vi "HOST_MAIN.vi"() -> ()   [LabVIEW 2023]
uses:
  RT/Type/Type_TCP_Cmd.ctl
  HOST_GLOBAL.vi
panel:
  in  "Bool_Exit":bool
  in  "Bool_main":bool
  in  "Bool_Config":bool
  out "Tab_Main":enum32{"Main", "Config"}(tab)
  out "Connected":i32(slide) scale=0.0..10.0
  out "R_GCP":sgl(slide) scale=0.0..100.0
  out "L_GCP":sgl(slide) scale=0.0..100.0
  in  "Save Data Path":path=path "C:/DataSave/Exosuit_FFM"
  out "TCP Connected":bool
  out "R_Velocity":sgl caption="[ kN ]" format="%#.4f"
  out "R_Position":sgl caption="[ kN ]" format="%#.4f"
  out "L_Velocity":sgl caption="[ kN ]" format="%#.4f"
  out "L_Position":sgl caption="[ kN ]" format="%#.4f"
  out "R_LOAD":sgl caption="[ N ]" format="%#.2f"
  out "L_LOAD":sgl caption="[ N ]" format="%#.2f"
  out "R_THIGH":sgl caption="[ kN ]"
  out "L_THIGH":sgl caption="[ kN ]"
  out "Pos_Chart":sgl[][](graph) caption="Motor Position"
  out "Load_Chart":sgl[][](graph) caption="LoadCell"
  out "IMU_Chart":sgl[][](graph) caption="IMU Sensor ROLL"
  in  "Bool_Auto_Stop":bool
  in  "Bool_Auto_Start":bool
  in  "Bool_SendConfig":bool
  in  "Param":T1={"Common"={"Velocity range"={"output high"=29.0, "output low"=-29.0}, "Vel_BasePos"=5, "Ref.Load_FindBase_L"=2.0, "Ref.Load_FindBase_R"=2.0, "Force_Peak"=150.0}, "Param_Left"={"L_기준값"=90.0, "L_검출값"=120.0, "L_End %"=42, "L_Onset %"=4, "L_Peak %"=28, "L_Pos"=0, "L_Offset"=0.0}, "Param_Right"={"R_기준값"=90.0, "R_검출값"=120.0, "R_End %"=42, "R_Onset %"=4, "R_Peak %"=28, "R_Pos"=0, "R_Offset"=0.0}}
  in  "탭 컨트롤":enum32{"Sensor", "Motor Status"}(tab)
  out "RIGHT":T2
  out "LEFT":T3
  in  "Port Number":u16
  in  "IP Address":string
  in  "Bool_Save_Config":bool
  # "실시간 보행 보조 로봇 모니터링 소프트웨어"
  # "Copyright ⓒ 2019 CAU all rights reserved"
  # "TCP Connection"
  # "TEST"
  # "DATA PATH"
  # "R - GCP [ % ]"
  # "L - GCP [ % ]"
  # "LOADCELL CONFIG"
  # "TEST PARAMETER"
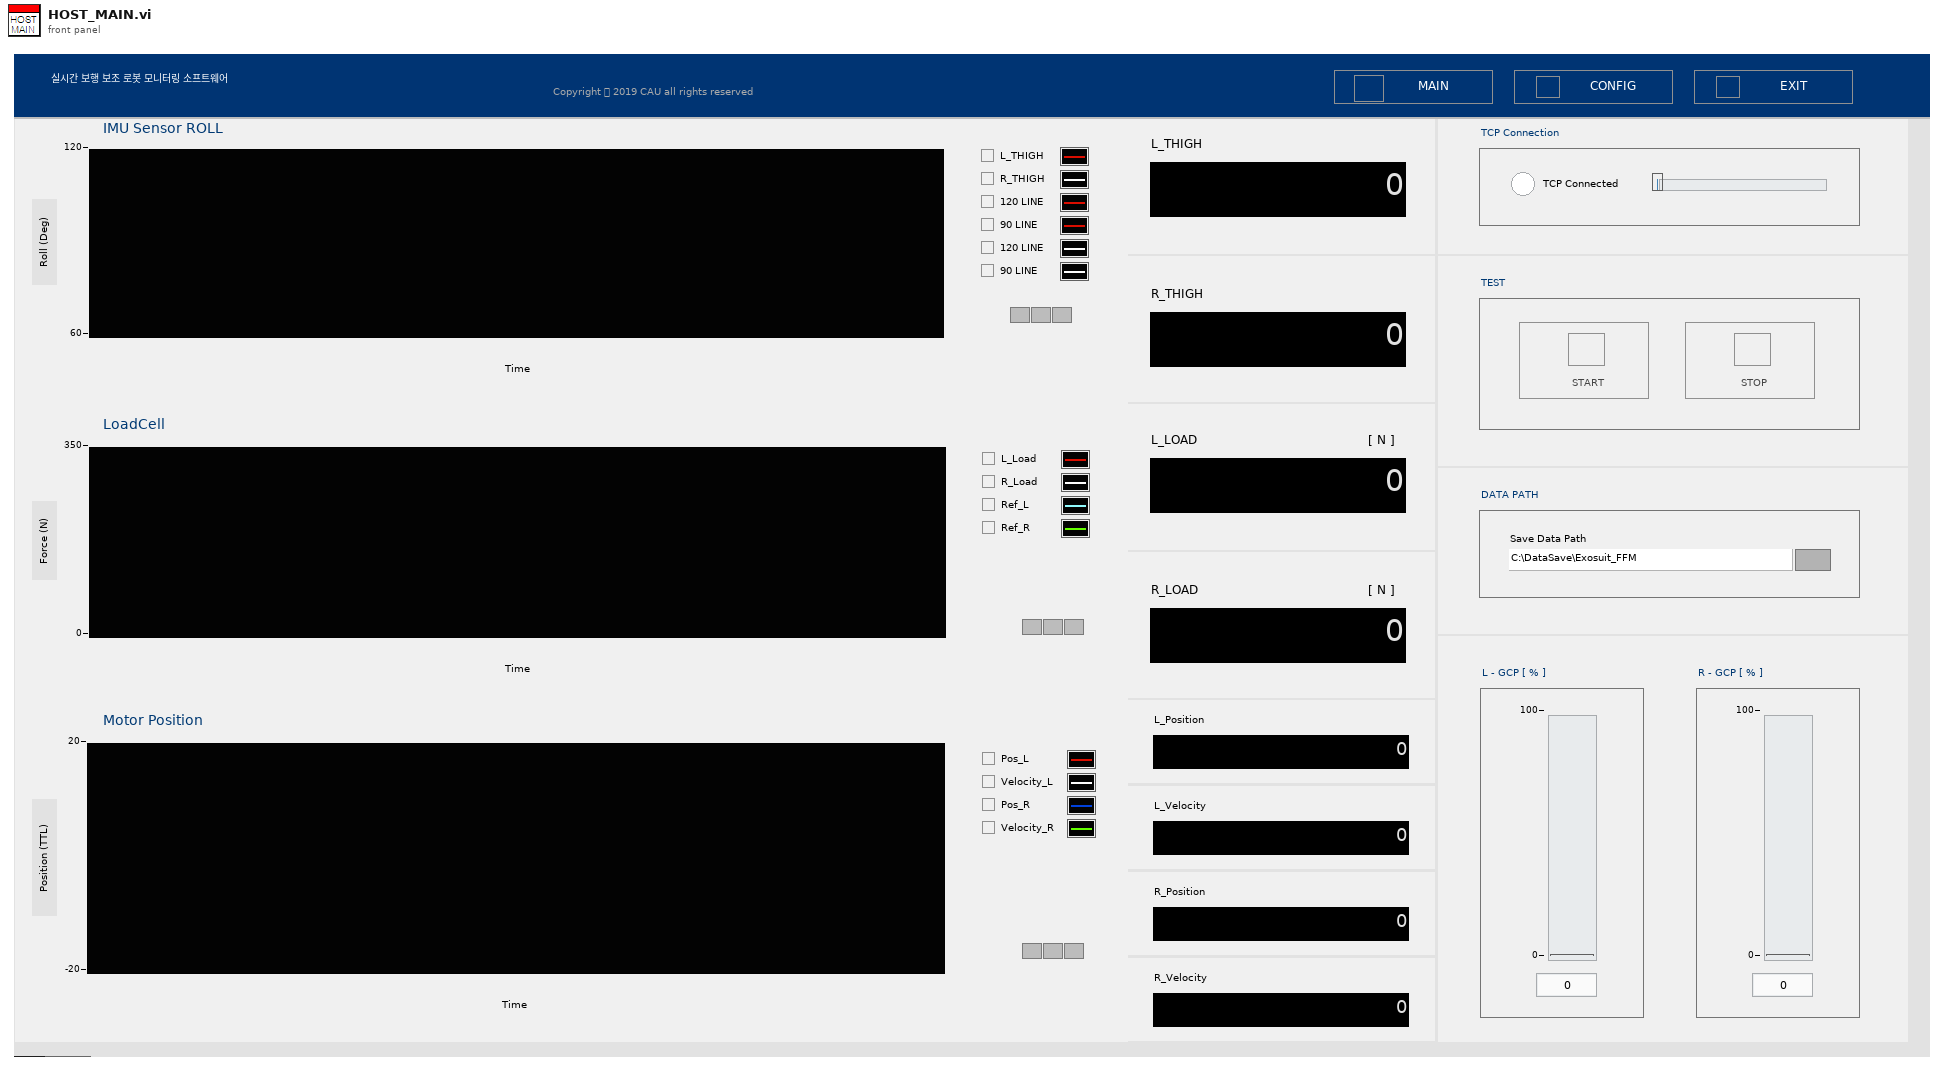
[diagram p1: front panel]
types:
  T1 = cluster{"Common":cluster{"Velocity range":cluster{"output high":dbl, "output low":dbl}, "Vel_BasePos":i32, "Ref.Load_FindBase_L":dbl, "Ref.Load_FindBase_R":dbl, "Force_Peak":dbl}, "Param_Left":cluster{"L_기준값":sgl, "L_검출값":sgl, "L_End %":i32, "L_Onset %":i32, "L_Peak %":i32, "L_Pos":i32, "L_Offset":sgl}, "Param_Right":cluster{"R_기준값":sgl, "R_검출값":sgl, "R_End %":i32, "R_Onset %":i32, "R_Peak %":i32, "R_Pos":i32, "R_Offset":sgl}}
  T2 = cluster{"Pos":sgl, "Velocity":sgl, "Loadcell":sgl, "IMU":sgl, "GCP":sgl}
  T3 = cluster{"Pos":sgl, "Velocity":sgl, "Loadcell_L":sgl, "IMU_L":sgl, "GCP_L":sgl}
  T4 = typedef "Type_TCP_Cmd.ctl" = enum16{"None", "Data", "Config", "Active"}
  T5 = cluster{"Velocity range":cluster{"output high":dbl, "output low":dbl}, "Enc counts to rad":dbl, "Vel_FindBase":i32, "Ref.Load_FindBase_L":dbl, "Ref.Load_FindBase_R":dbl, "Pos_L.Base":dbl, "Pos_R.Base":dbl, "Force_Peak":dbl, "Clt_Param":cluster{"Clt_Param_L":cluster{"기준값":sgl, "검출값":sgl, "End %":i32, "Onset %":i32, "Peak %":i32, "Pos":i32, "Offset":sgl}, "Clt_Param_R":cluster{"기준값":sgl, "검출값":sgl, "End %":i32, "Onset %":i32, "Peak %":i32, "Pos":i32, "Offset":sgl}}}
  T6 = cluster{"Sensor_Data":sgl[], "Status_L":cluster{"Ready to switch on":bool, "Switched on":bool, "Operation enable":bool, "Fault":bool, "Voltage enable":bool, "Quick stop":bool, "Switch on disable":bool, "not used (warning)":bool, "Offset current measured":bool, "Remote":bool, "Operation mode specific":bool, "Internal limit active":bool, "Operation mode specific":bool, "Operation mode specific":bool, "Refresh cycle of power stage":bool, "Position referenced to home position":bool}, "Status_R":cluster{"Ready to switch on":bool, "Switched on":bool, "Operation enable":bool, "Fault":bool, "Voltage enable":bool, "Quick stop":bool, "Switch on disable":bool, "not used (warning)":bool, "Offset current measured":bool, "Remote":bool, "Operation mode specific":bool, "Internal limit active":bool, "Operation mode specific":bool, "Operation mode specific":bool, "Refresh cycle of power stage":bool, "Position referenced to home position":bool}, "D_Current_L":i32, "D_Current_R":i32, "A_Current_L":sgl, "A_Current_R":sgl, "D_Vel_L":sgl, "D_Vel_R":sgl, "A_Velocity_L":sgl, "A_Velocity_R":sgl, "A_Pos_L":sgl, "A_Pos_R":sgl, "Force_Reference":sgl[], "GCP_L":sgl, "GCP_R":sgl, "Wire_pull_L":bool, "Wire_pull_R":bool}
  T7 = cluster{"Pos":sgl, "Velocity":sgl, "Force":sgl, "Roll":sgl, "GCP":sgl}
  T8 = cluster{"기준값":sgl, "검출값":sgl, "End %":i32, "Onset %":i32, "Peak %":i32, "Pos":i32, "Offset":sgl}
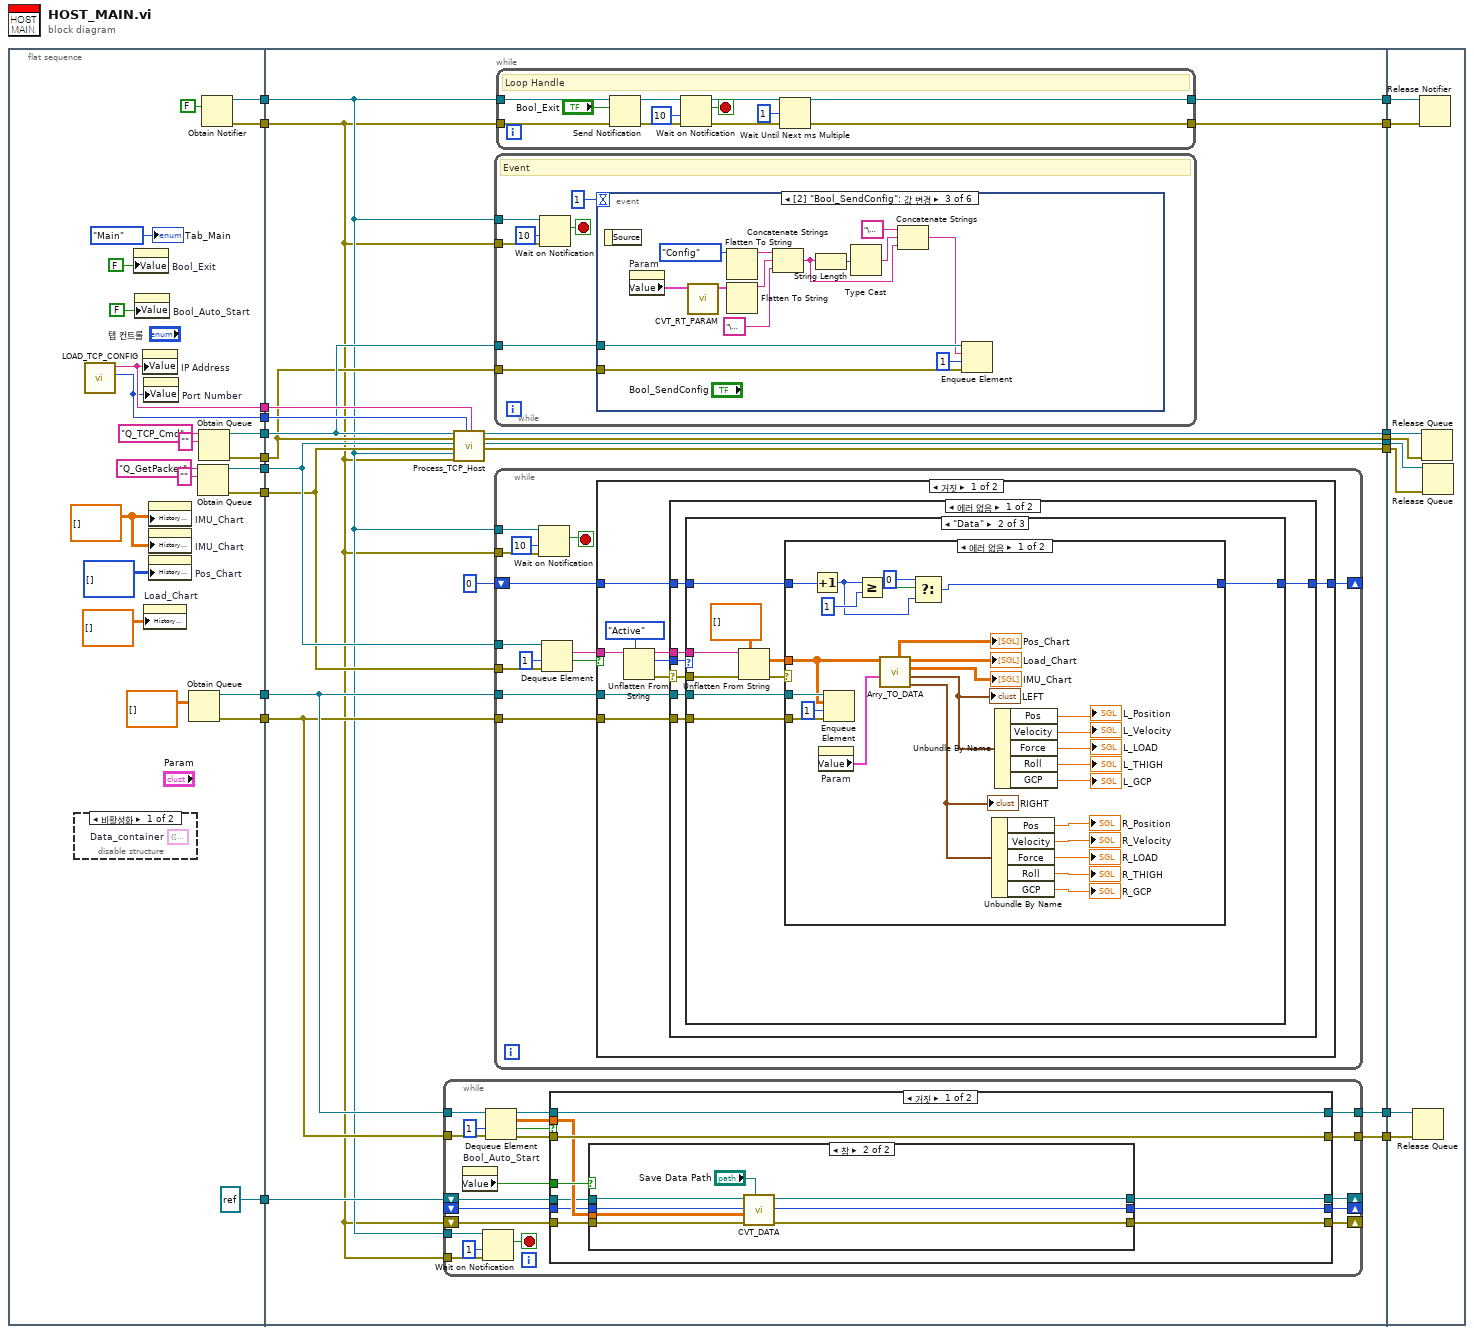
[diagram p0: block diagram]
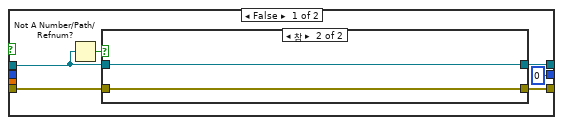
[diagram p3: hidden frame]
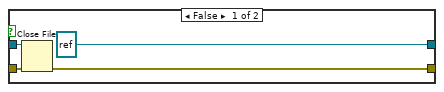
[diagram p4: hidden frame]
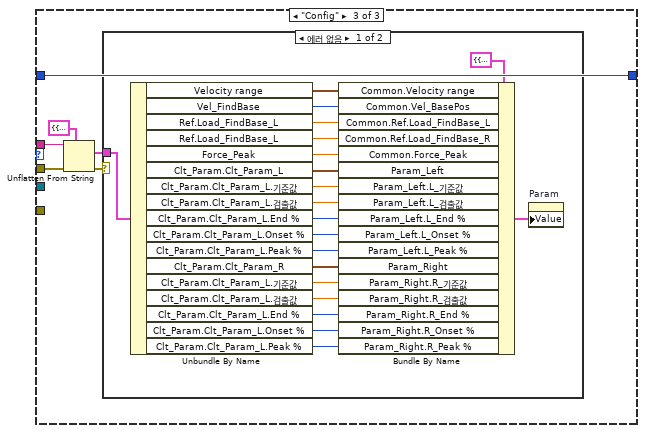
[diagram p8: hidden frame]
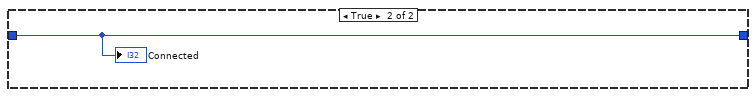
[diagram p11: hidden frame]
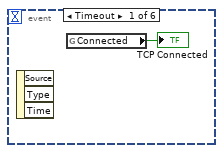
[diagram p12: hidden frame]
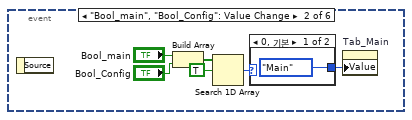
[diagram p13: hidden frame]
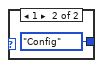
[diagram p14: hidden frame]
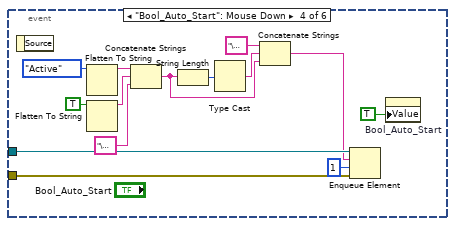
[diagram p15: hidden frame]
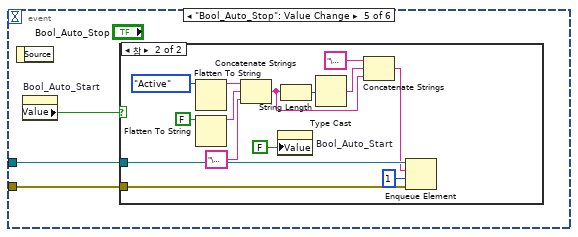
[diagram p16: hidden frame]
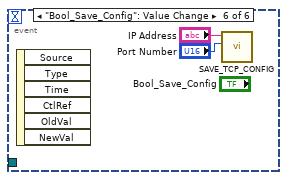
[diagram p18: hidden frame]
diagram:
  n1 = flat-sequence {
    tunnel: [w41] -> w19
    tunnel: [w40] -> w18
    tunnel: [w35] -> w17
    tunnel: [w34] -> w16
    tunnel: [w33] -> w15
    tunnel: [w32] -> w14
    tunnel: [w22] -> w13
    tunnel: [w23] -> w12
    tunnel: [w28] -> w11
    tunnel: [w27] -> w10
    tunnel: [refnum<file> refnum ("참조 번호 출력")] -> w9
    tunnel: w19 -> [w49]
    tunnel: w18 -> [w48]
    tunnel: [w62] -> w8
    tunnel: [w61] -> w7
    tunnel: w17 -> [w53]
    tunnel: w16 -> [w52]
    tunnel: w15 -> [w51]
    tunnel: w14 -> [w50]
    tunnel: w13 -> [w54]
    tunnel: w12 -> [w55]
    tunnel: [w47] -> w6
    tunnel: [w46] -> w5
    tunnel: [w45] -> w4
    tunnel: [w44] -> w3
    tunnel: w11 -> [w60]
    tunnel: w10 -> [w59]
    tunnel: [w58] -> w2
    tunnel: [w57] -> w1
    tunnel: w9 -> [w56]
    tunnel: w8 -> [w292]
    tunnel: w7 -> [w291]
    tunnel: w6 -> [w290]
    tunnel: w5 -> [w289]
    tunnel: w4 -> [w288]
    tunnel: w3 -> [w287]
    tunnel: w2 -> [w286]
    tunnel: w1 -> [w285]
    frame #0 {
      w25 = sgl[][] [] ("히스토리 데이터")
      n2 = disable-structure shown="비활성화" {
        frame Disabled {
          (unwired) T6 {"Sensor_Data"=[], "Status_L"={"Ready to switch on"=TRUE, "Switched on"=TRUE, "Operation enable"=TRUE, "Fault"=FALSE, "Voltage enable"=TRUE, "Quick stop"=TRUE, "Switch on disable"=FALSE, "not used (warning)"=FALSE, "Offset current measured"=FALSE, "Remote"=TRUE, "Operation mode specific"=TRUE, "Internal limit active"=FALSE, "Operation mode specific"=FALSE, "Operation mode specific"=FALSE, "Refresh cycle of power stage"=FALSE, "Position referenced to home position"=FALSE}, "Status_R"={"Ready to switch on"=TRUE, "Switched on"=TRUE, "Operation enable"=TRUE, "Fault"=FALSE, "Voltage enable"=TRUE, "Quick stop"=TRUE, "Switch on disable"=FALSE, "not used (warning)"=FALSE, "Offset current measured"=FALSE, "Remote"=TRUE, "Operation mode specific"=TRUE, "Internal limit active"=FALSE, "Operation mode specific"=FALSE, "Operation mode specific"=FALSE, "Refresh cycle of power stage"=FALSE, "Position referenced to home position"=FALSE}, "D_Current_L"=0, "D_Current_R"=0, "A_Current_L"=0.0, "A_Current_R"=0.0, "D_Vel_L"=0.0, "D_Vel_R"=0.0, "A_Velocity_L"=0.0, "A_Velocity_R"=0.0, "A_Pos_L"=0.0, "A_Pos_R"=0.0, "Force_Reference"=[0.0, 0.0], "GCP_L"=0.0, "GCP_R"=0.0, "Wire_pull_L"=FALSE, "Wire_pull_R"=FALSE}  # Data_container
        }
        frame Enabled {
        }
      }
      n3 = call "LOAD_TCP_CONFIG.vi"() -> ("PortNumber"=w22:u16, "IP Addr"=w23:string)  [unwired: 10 in]
      n4 = property on="Bool_Exit" class="Bool (엄격한)"("Value"=FALSE ("Bool_Exit")) -> ()  [unwired: 2 in, 2 out]
      n5 = property on="Bool_Auto_Start" class="Bool (엄격한)"("Value"=FALSE ("Bool_Auto_Start")) -> ()  [unwired: 2 in, 2 out]
      n6 = property on="IP Address" class="Str"("Value"=w23) -> ()  [unwired: 2 in, 2 out]
      n7 = property on="Port Number" class="DigNum (엄격한)"("Value"=w22) -> ()  [unwired: 2 in, 2 out]
      n8 = property on="Load_Chart" class="WFChart (엄격한)"("History Data"=sgl[][] [] ("히스토리 데이터")) -> ()  [unwired: 2 in, 2 out]
      n9 = property on="IMU_Chart" class="WFChart (엄격한)"("History Data"=w25) -> ()  [unwired: 2 in, 2 out]
      n10 = property on="IMU_Chart" class="WFChart (엄격한)"("History Data"=w25) -> ()  [unwired: 2 in, 2 out]
      n11 = property on="Pos_Chart" class="WFChart (엄격한)"("History Data"=i32[][] [] ("히스토리 데이터")) -> ()  [unwired: 2 in, 2 out]
      n12 = Obtain Queue(element data type=sgl[][] []) -> (queue out=w28:refnum<queue>, error out=w27:errorcluster)  [unwired: 4 in, 1 out]
      n13 = Obtain Queue(name (unnamed)="Q_GetPacket" ("이름(이름없음)"), element data type="") -> (queue out=w33:refnum<queue>, error out=w32:errorcluster)  [unwired: 3 in, 1 out]
      n14 = Obtain Queue(name (unnamed)="Q_TCP_Cmd" ("이름(이름없음)"), element data type="") -> (queue out=w35:refnum<queue>, error out=w34:errorcluster)  [unwired: 3 in, 1 out]
      n15 = Obtain Notifier(notification data type=FALSE) -> (notifier out=w41:refnum<notifier>, error out=w40:errorcluster)  [unwired: 3 in, 1 out]
      "Tab_Main" <- enum32{"Main", "Config"}."Main" ("Tab_Main")
    }
    frame #1 {
      n16 = while {
        tunnel: w60 -> [w80]
        tunnel: w59 -> [w79]
        tunnel: w49 -> [w78]
        tunnel: w48 -> [w77]
        tunnel: [w73] -> w58
        tunnel: [w70] -> w57
        shift-right: [w67] -> _
        shift-left: w56 -> [w68]
        shift-right: [w66] -> _
        shift-left: w48 -> [w65]
        shift-right: [w64] -> _
        shift-left: _ -> [w63]
        stop <- w76 stop-if-true
        n17 = property on="Bool_Auto_Start" class="Bool (엄격한)"() -> ("Value"=w69:bool)  [unwired: 2 in, 2 out]
        n18 = Wait on Notification(notifier=w78, timeout in ms (-1)=1 ("타임아웃(ms) (-1)"), error in (no error)=w77) -> (notification=w76:bool)  [unwired: 1 in, 3 out]
        n19 = Dequeue Element(queue=w80, timeout in ms (-1)=1 ("타임아웃(ms) (-1)"), error in (no error)=w79) -> (queue out=w72:refnum<queue>, element=w74:sgl[][], timed out?=w75:bool, error out=w71:errorcluster)
        n20 = case shown="거짓" w75 {
          tunnel: w74 -> [w89 _]
          tunnel: [w92 w117] -> w73
          tunnel: w72 -> [w92 w117]
          tunnel: w71 -> [w91 w116]
          tunnel: [w91 w116] -> w70
          tunnel: w69 -> [w90 _]
          tunnel: w68 -> [w88 w115]
          tunnel: [w87 w115] -> w67
          tunnel: [w86 w114] -> w66
          tunnel: w65 -> [w85 w114]
          tunnel: [w84 w113] -> w64
          tunnel: w63 -> [w83 w113]
          frame False {
            n21 = case shown="참" w90 {
              tunnel: w89 -> [_ w107]
              tunnel: w88 -> [w96 w111]
              tunnel: [w94 w112] -> w87
              tunnel: [w95 w109] -> w86
              tunnel: w85 -> [w97 w110]
              tunnel: [u32 0 ("10_Count_Out") w106] -> w84
              tunnel: w83 -> [_ w105]
              frame False {
                n22 = Not A Number/Path/Refnum?(number/path/refnum=w96) -> (NaN/Path/Refnum?=w98:bool)
                n23 = case shown="참" w98 {
                  tunnel: w97 -> [w101 w104]
                  tunnel: w96 -> [w102 w103]
                  tunnel: [w99 w104] -> w95
                  tunnel: [refnum<file> refnum ("참조 번호 출력") w103] -> w94
                  frame False {
                    n24 = Close File(refnum=w102, error in=w101) -> (error out=w99:errorcluster)  [unwired: 1 out]
                  }
                  frame True {
                  }
                }
              }
              frame True {
                n25 = call "CVT_DATA.vi"("경로"="Save Data Path", "error in"=w110, "DATA"=w107, "10_Count_In"=w105, "ref_file_in"=w111) -> ("error out"=w109:errorcluster, "10_Count_Out"=w106:u32, "ref_file_Out"=w112:refnum<file>)  [unwired: 4 in]
              }
            }
          }
          frame True {
          }
        }
      }
      n26 = call "Process_TCP_Host.vi"("Q_TCP_Cmd_IN"=w53, "Q_TCP_Cmd_Err_IN"=w52, "Q_GetPacket_IN"=w51, "Q_GetPacket_Err_IN"=w50, "Notifier_IN"=w49, "Notifier_Err_IN"=w48, "PortNumber"=w54, "IP Addr"=w55) -> ("Q_TCP_Cmd_OUT"=w47:refnum<queue>, "Q_TCP_Cmd_Err_OUT"=w46:errorcluster, "Q_GetPacket_OUT"=w45:refnum<queue>, "Q_GetPacket_Err_OUT"=w44:errorcluster)  [unwired: 8 in]
      n27 = while {
        tunnel: w49 -> [w217]
        tunnel: w48 -> [w216]
        tunnel: w53 -> [w213]
        tunnel: w52 -> [w212]
        stop <- w214 stop-if-true
        # "Event"
        n28 = Wait on Notification(notifier=w217, timeout in ms (-1)=10 ("타임아웃(ms) (-1)"), error in (no error)=w216) -> (notification=w214:bool)  [unwired: 1 in, 3 out]
        n29 = event shown="[2] \"Bool_SendConfig\": 값 변경" {
          selector: _ -> [_ _ _ _ _ _]
          dyn-events: _ -> [_ _ _ _ _ _]
          timeout: 1 -> [_ _ _ _ _ _]
          tunnel: w213 -> [_ _ w233 w247 w258 _]
          tunnel: w212 -> [_ _ w232 w246 w257 _]
          event Timeout {
            n30 = event-data() -> ()  [unwired: 1 in, 3 out]
            n31 = global read "HOST_GLOBAL.vi" "Connected"() -> (→"TCP Connected":bool)
          }
          event "Bool_main", "Bool_Config": Value Change {
            n32 = event-data() -> ()  [unwired: 1 in, 1 out]
            n33 = Build Array("Bool_main", "Bool_Config") -> (w223:bool[])
            n34 = Search 1D Array(1D array=w223, element=TRUE ("원소")) -> (index of element=w221:i32)  [unwired: 1 in]
            n35 = case shown="0, 기본" w221 {
              tunnel: [enum32{"Main", "Config"}."Main" ("Tab_Main") enum32{"Main", "Config"}."Config" ("Tab_Main")] -> w220
              frame 0, Default {
              }
              frame 1 {
              }
            }
            n36 = property on="Tab_Main" class="TabCtl (엄격한)"("Value"=w220) -> ()  [unwired: 2 in, 2 out]
          }
          event "Bool_SendConfig": Value Change {
            n37 = event-data() -> ()  [unwired: 1 in, 1 out]
            n38 = property on="Param" class="Clust (엄격한)"() -> ("Value"=w228:T1)  [unwired: 2 in, 2 out]
            n39 = call "CVT_RT_PARAM.vi"("Param"=w228) -> ("RT_Config"=w229:T5)  [unwired: 10 in]
            n40 = Flatten To String(anything=Type_TCP_Cmd."Config") -> (data string=w240:string)  [unwired: 3 in, 2 out]
            n41 = Flatten To String(anything=w229) -> (data string=w239:string)  [unwired: 3 in, 2 out]
            n42 = Concatenate Strings(w240, w239, "\u0003" ("문자열")) -> (w235:string)
            n43 = String Length(string=w235) -> (length=w238:i32)
            n44 = Type Cast(x=w238) -> (*(type *) &x=w237:string)  [unwired: 1 in]
            n45 = Concatenate Strings("\u0002" ("문자열"), w237, w235) -> (w230:string)
            n46 = Enqueue Element(queue=w233, element=w230, timeout in ms (-1)=1 ("타임아웃(ms) (-1)"), error in (no error)=w232) -> ()  [unwired: 3 out]
          }
          event "Bool_Auto_Start": Mouse Down {
            n47 = event-data() -> ()  [unwired: 1 in, 1 out]
            n48 = Flatten To String(anything=Type_TCP_Cmd."Active") -> (data string=w254:string)  [unwired: 3 in, 2 out]
            n49 = Flatten To String(anything=TRUE) -> (data string=w253:string)  [unwired: 3 in, 2 out]
            n50 = Concatenate Strings(w254, w253, "\u0003" ("문자열")) -> (w249:string)
            n51 = String Length(string=w249) -> (length=w252:i32)
            n52 = Type Cast(x=w252) -> (*(type *) &x=w251:string)  [unwired: 1 in]
            n53 = Concatenate Strings("\u0002" ("문자열"), w251, w249) -> (w244:string)
            n54 = Enqueue Element(queue=w247, element=w244, timeout in ms (-1)=1 ("타임아웃(ms) (-1)"), error in (no error)=w246) -> ()  [unwired: 3 out]
            n55 = property on="Bool_Auto_Start" class="Bool (엄격한)"("Value"=TRUE ("Bool_Auto_Start")) -> ()  [unwired: 2 in, 2 out]
          }
          event "Bool_Auto_Stop": Value Change {
            n56 = event-data() -> ()  [unwired: 1 in, 1 out]
            n57 = property on="Bool_Auto_Start" class="Bool (엄격한)"() -> ("Value"=w256:bool)  [unwired: 2 in, 2 out]
            n58 = case shown="참" w256 {
              tunnel: w258 -> [_ w264]
              tunnel: w257 -> [_ w263]
              frame False {
              }
              frame True {
                n59 = Flatten To String(anything=Type_TCP_Cmd."Active") -> (data string=w271:string)  [unwired: 3 in, 2 out]
                n60 = Flatten To String(anything=FALSE) -> (data string=w270:string)  [unwired: 3 in, 2 out]
                n61 = Concatenate Strings(w271, w270, "\u0003" ("문자열")) -> (w266:string)
                n62 = property on="Bool_Auto_Start" class="Bool (엄격한)"("Value"=FALSE ("Bool_Auto_Start")) -> ()  [unwired: 2 in, 2 out]
                n63 = String Length(string=w266) -> (length=w269:i32)
                n64 = Type Cast(x=w269) -> (*(type *) &x=w268:string)  [unwired: 1 in]
                n65 = Concatenate Strings("\u0002" ("문자열"), w268, w266) -> (w261:string)
                n66 = Enqueue Element(queue=w264, element=w261, timeout in ms (-1)=1 ("타임아웃(ms) (-1)"), error in (no error)=w263) -> ()  [unwired: 3 out]
              }
            }
          }
          event "Bool_Save_Config": Value Change {
            n67 = event-data() -> ()  [unwired: 1 in, 6 out]
            n68 = call "SAVE_TCP_CONFIG.vi"("PortNumber"="Port Number", "IP Addr"="IP Address") -> ()  [unwired: 9 in, 1 out]
          }
        }
      }
      n69 = while {
        tunnel: w49 -> [w125]
        tunnel: w48 -> [w124]
        tunnel: w51 -> [w118]
        tunnel: w50 -> [w130]
        tunnel: w60 -> [w122]
        tunnel: w59 -> [w121]
        shift-right: [w119] -> _
        shift-left: 0 -> [w120]
        stop <- w123 stop-if-true
        n70 = Wait on Notification(notifier=w125, timeout in ms (-1)=10 ("타임아웃(ms) (-1)"), error in (no error)=w124) -> (notification=w123:bool)  [unwired: 1 in, 3 out]
        n71 = Dequeue Element(queue=w118, timeout in ms (-1)=1 ("타임아웃(ms) (-1)"), error in (no error)=w130) -> (element=w127:string, timed out?=w128:bool)  [unwired: 2 out]
        n72 = case shown="거짓" w128 {
          tunnel: w127 -> [w138 _]
          tunnel: w122 -> [w134 _]
          tunnel: w121 -> [w133 _]
          tunnel: w120 -> [w132 w211]
          tunnel: [w131 w211] -> w119
          frame False {
            n73 = Unflatten From String(type=Type_TCP_Cmd."Active" ("Type_TCP_Cmd"), binary string=w138) -> (rest of the binary string=w135:string, value=w136:T4, error out=w137:errorcluster)  [unwired: 3 in]
            n74 = case shown="에러 없음" w137 {
              selector: w137 -> [w144 _]
              tunnel: w136 -> [w146 _]
              tunnel: w135 -> [w145 _]
              tunnel: w134 -> [w143 _]
              tunnel: w133 -> [w142 _]
              tunnel: w132 -> [w141 w210]
              tunnel: [w140 w210] -> w131
              frame No Error {
                n75 = case shown="\"Data\"" w146 {
                  tunnel: w145 -> [_ w156 w189]
                  tunnel: w144 -> [_ w155 w188]
                  tunnel: w143 -> [_ w152 _]
                  tunnel: w142 -> [_ w151 _]
                  tunnel: w141 -> [w147 w150 w185]
                  tunnel: [w147 w149 w185] -> w140
                  frame "None", Default {
                  }
                  frame "Data" {
                    n76 = Unflatten From String(type=sgl[][] [], binary string=w156, error in (no error)=w155) -> (value=w153:sgl[][], error out=w154:errorcluster)  [unwired: 2 in, 1 out]
                    n77 = case shown="에러 없음" w154 {
                      tunnel: w153 -> [w177 _]
                      tunnel: w152 -> [w182 _]
                      tunnel: w151 -> [w181 _]
                      tunnel: w150 -> [w176 w183]
                      tunnel: [w171 w183] -> w149
                      frame No Error {
                        n78 = Increment(x=w176) -> (x+1=w173:i32)
                        n79 = property on="Param" class="Clust (엄격한)"() -> ("Value"=w157:T1)  [unwired: 2 in, 2 out]
                        n80 = Enqueue Element(queue=w182, element=w177, timeout in ms (-1)=1 ("타임아웃(ms) (-1)"), error in (no error)=w181) -> ()  [unwired: 3 out]
                        n81 = Greater Or Equal?(x=w173, y=1) -> (x >= y?=w174:bool)
                        n82 = call "Arry_TO_DATA.vi"("Param"=w157, "DATA"=w177) -> ("RIGHT"=w165:T7, "LEFT"=w158:T7, "IMU"=→"IMU_Chart":sgl[][], "LoadCell"=→"Load_Chart":sgl[][], "PosVel"=→"Pos_Chart":sgl[][])  [unwired: 5 in]
                        "LEFT" <- w158
                        "RIGHT" <- w165
                        n83 = Select(t=0, s=w174, f=w173) -> (s? t:f=w171:i32)
                        n84 = Unbundle By Name(w165) -> ("Pos"=→"R_Position":sgl, "Velocity"=→"R_Velocity":sgl, "Force"=→"R_LOAD":sgl, "Roll"=→"R_THIGH":sgl, "GCP"=→"R_GCP":sgl)
                        n85 = Unbundle By Name(w158) -> ("Pos"=→"L_Position":sgl, "Velocity"=→"L_Velocity":sgl, "Force"=→"L_LOAD":sgl, "Roll"=→"L_THIGH":sgl, "GCP"=→"L_GCP":sgl)
                      }
                      frame Error {
                      }
                    }
                  }
                  frame "Config" {
                    n86 = Unflatten From String(type=T5 {"Velocity range"={"output high"=0.0, "output low"=0.0}, "Enc counts to rad"=0.0, "Vel_FindBase"=0, "Ref.Load_FindBase_L"=0.0, "Ref.Load_FindBase_R"=0.0, "Pos_L.Base"=0.0, "Pos_R.Base"=0.0, "Force_Peak"=0.0, "Clt_Param"={"Clt_Param_L"={"기준값"=0.0, "검출값"=0.0, "End %"=0, "Onset %"=0, "Peak %"=0, "Pos"=0, "Offset"=0.0}, "Clt_Param_R"={"기준값"=0.0, "검출값"=0.0, "End %"=0, "Onset %"=0, "Peak %"=0, "Pos"=0, "Offset"=0.0}}} ("Param 2"), binary string=w189, error in (no error)=w188) -> (value=w187:T5, error out=w186:errorcluster)  [unwired: 2 in, 1 out]
                    n87 = case shown="에러 없음" w186 {
                      tunnel: w187 -> [w209 _]
                      frame No Error {
                        n88 = Unbundle By Name(w209) -> ("Velocity range"=w208:cluster{"output high":dbl, "output low":dbl}, "Vel_FindBase"=w207:i32, "Ref.Load_FindBase_L"=w206:dbl, "Ref.Load_FindBase_L"=w205:dbl, "Force_Peak"=w193:dbl, "Clt_Param.Clt_Param_L"=w194:T8, "Clt_Param.Clt_Param_L.기준값"=w204:sgl, "Clt_Param.Clt_Param_L.검출값"=w203:sgl, "Clt_Param.Clt_Param_L.End %"=w202:i32, "Clt_Param.Clt_Param_L.Onset %"=w201:i32, "Clt_Param.Clt_Param_L.Peak %"=w192:i32, "Clt_Param.Clt_Param_R"=w191:T8, "Clt_Param.Clt_Param_L.기준값"=w200:sgl, "Clt_Param.Clt_Param_L.검출값"=w199:sgl, "Clt_Param.Clt_Param_L.End %"=w198:i32, "Clt_Param.Clt_Param_L.Onset %"=w197:i32, "Clt_Param.Clt_Param_L.Peak %"=w190:i32)
                        n89 = Bundle By Name(cluster=T1 {"Common"={"Velocity range"={"output high"=29.0, "output low"=-29.0}, "Vel_BasePos"=5, "Ref.Load_FindBase_L"=2.0, "Ref.Load_FindBase_R"=2.0, "Force_Peak"=150.0}, "Param_Left"={"L_기준값"=90.0, "L_검출값"=120.0, "L_End %"=42, "L_Onset %"=4, "L_Peak %"=28, "L_Pos"=0, "L_Offset"=0.0}, "Param_Right"={"R_기준값"=90.0, "R_검출값"=120.0, "R_End %"=42, "R_Onset %"=4, "R_Peak %"=28, "R_Pos"=0, "R_Offset"=0.0}} ("Param 2"), "Common.Velocity range"=w208, "Common.Vel_BasePos"=w207, "Common.Ref.Load_FindBase_L"=w206, "Common.Ref.Load_FindBase_R"=w205, "Common.Force_Peak"=w193, "Param_Left"=w194, "Param_Left.L_기준값"=w204, "Param_Left.L_검출값"=w203, "Param_Left.L_End %"=w202, "Param_Left.L_Onset %"=w201, "Param_Left.L_Peak %"=w192, "Param_Right"=w191, "Param_Right.R_기준값"=w200, "Param_Right.R_검출값"=w199, "Param_Right.R_End %"=w198, "Param_Right.R_Onset %"=w197, "Param_Right.R_Peak %"=w190) -> (w195:T1)
                        n90 = property on="Param" class="Clust (엄격한)"("Value"=w195) -> ()  [unwired: 2 in, 2 out]
                      }
                      frame Error {
                      }
                    }
                  }
                }
              }
              frame Error {
              }
            }
          }
          frame True {
            "Connected" <- w211
          }
        }
      }
      n91 = while "While 루프" {
        tunnel: w49 -> [w283]
        tunnel: w48 -> [w282]
        tunnel: [w279] -> w62
        tunnel: [w278] -> w61
        stop <- w277 stop-if-true
        # "Loop Handle"
        n92 = Send Notification(notification="Bool_Exit", notifier=w283, error in (no error)=w282) -> (notifier out=w281:refnum<notifier>, error out=w280:errorcluster)
        n93 = Wait on Notification(notifier=w281, timeout in ms (-1)=10 ("타임아웃(ms) (-1)"), error in (no error)=w280) -> (notifier out=w279:refnum<notifier>, notification=w277:bool, error out=w278:errorcluster)  [unwired: 1 in, 1 out]
        n94 = Wait Until Next ms Multiple(millisecond multiple=u32 1 ("대기 시간(ms)")) -> ()  [unwired: 1 out]
      }
    }
    frame #2 {
      n95 = Release Queue(queue=w286, error in (no error)=w285) -> ()  [unwired: 1 in, 3 out]
      n96 = Release Notifier(notifier=w292, error in (no error)=w291) -> ()  [unwired: 1 in, 3 out]
      n97 = Release Queue(queue=w290, error in (no error)=w289) -> ()  [unwired: 1 in, 3 out]
      n98 = Release Queue(queue=w288, error in (no error)=w287) -> ()  [unwired: 1 in, 3 out]
    }
  }
